vi "总磷总氮测量数据储存.vi"   [LabVIEW 2016, in "斯坦道总磷.lvlib"]
types:
  T1 = enum16{"水样测试", "标样核查", "跨度核查", "零点核查", "加标回收", "空白测试", "平行样"}
  T2 = cluster{"时间标识":timestamp, "测量模式":enum16{"维护数据", "水样测试", "标样核查", "零点核查", "跨度核查", "空白测试", "平行样测试", "加标回收", "空白校准", "标样校准", "初始化（清洗）", "快捷测试"}, "数据标记表":string, "监测值":sgl, "单位":u16, "数据标识":string, "因子编码":u32, "标样参考值":sgl, "F0":sgl, "F1":sgl, "F2":sgl, "F3":sgl, "F4":sgl, "F5":sgl, "F6":sgl, "F7":sgl, "X":sgl, "温度":sgl, "湿度":sgl, "量程标识":string, "SN":string, "跨度值":sgl, "X1":sgl}
  T3 = enum16{"维护数据", "水样测试", "标样核查", "零点核查", "跨度核查", "空白测试", "平行样测试", "加标回收", "空白校准", "标样校准", "初始化（清洗）", "快捷测试"}
  T4 = enum16{"维护数据", "水样测试", "标样核查", "零点核查", "跨度核查", "空白测试", "平行样测试", "加标回收", "空白校准", "标样校准", "初始化（清洗）"}
  T5 = cluster{"系统时间":timestamp, "工作状态":u16, "测量模式":enum16{"待机", "连续模式", "周期模式", "定点模式", "受控模式", "手动模式"}, "告警代码":u16, "故障代码":u16, "日志代码":u16, "软件版本":u16, "F0":sgl, "F1":sgl, "F2":sgl, "F3":sgl, "T":sgl, "H":sgl, "id":u16, "flowid":u16, "量程":u16, "总磷控温温度1":sgl, "营养盐控温温度2":sgl, "ADC":sgl}
  T6 = cluster{"运行模式":enum16{"维护模式", "常规模式", "应急模式", "质控模式"}, "质控频次":enum16{"关闭", "每天", "星期一", "星期二", "星期三", "星期四", "星期五", "星期六", "星期日"}, "空白核查时间":u16, "跨度核查时间":u16, "24H周期设置":bool[]}
  T7 = cluster{"因子编码":u32, "单位":u16, "标样参考值":sgl, "水样数据时间":timestamp, "水样实测值":sgl, "水样数据标识":string, "标样数据时间":timestamp, "标样实测值":sgl, "标样数据标识":string, "空白数据时间":timestamp, "空白实测值":sgl, "空白数据标识":string, "零点核查数据时间":timestamp, "零点核查实测值":sgl, "零点核查数据标识":string, "跨度核查数据时间":timestamp, "跨度核查实测值":sgl, "跨度核查数据标识":string, "加标回收数据时间":timestamp, "加标回收实测值":sgl, "加标回收数据标识":string, "平行样数据时间":timestamp, "平行样实测值":sgl, "平行样数据标识":string, "F0":sgl, "F1":sgl, "F2":sgl, "F3":sgl, "F4":sgl, "F5":sgl, "F6":sgl, "F7":sgl, "温度":sgl, "湿度":sgl, "X值":sgl, "fidrange":u16, "X1值":sgl}[]
  T8 = cluster{"因子编码":u32, "单位":u16, "标样参考值":sgl, "水样数据时间":timestamp, "水样实测值":sgl, "水样数据标识":string, "标样数据时间":timestamp, "标样实测值":sgl, "标样数据标识":string, "空白数据时间":timestamp, "空白实测值":sgl, "空白数据标识":string, "零点核查数据时间":timestamp, "零点核查实测值":sgl, "零点核查数据标识":string, "跨度核查数据时间":timestamp, "跨度核查实测值":sgl, "跨度核查数据标识":string, "加标回收数据时间":timestamp, "加标回收实测值":sgl, "加标回收数据标识":string, "平行样数据时间":timestamp, "平行样实测值":sgl, "平行样数据标识":string, "F0":sgl, "F1":sgl, "F2":sgl, "F3":sgl, "F4":sgl, "F5":sgl, "F6":sgl, "F7":sgl, "温度":sgl, "湿度":sgl, "X值":sgl, "fidrange":u16, "X1值":sgl}
  T9 = cluster{"总磷跨度值":dbl, "总磷零点标准液浓度":dbl, "总磷跨度标准液浓度":dbl, "总磷标准液标准浓度":dbl, "总氮跨度值":dbl, "总氮零点标准液浓度":dbl, "总氮跨度标准液浓度":dbl, "总氮标准液标准浓度":dbl, "COD跨度值":dbl, "COD零点标准液浓度":dbl, "COD跨度标准液浓度":dbl, "COD标准液标准浓度":dbl, "氨氮跨度值":dbl, "氨氮零点标准液浓度":dbl, "氨氮跨度标准液浓度":dbl, "氨氮标准液标准浓度":dbl, "磷酸盐跨度值":dbl, "磷酸盐零点标准液浓度":dbl, "磷酸盐跨度标准液浓度":dbl, "磷酸盐标准液标准浓度":dbl, "硝氮跨度值":dbl, "硝氮零点标准液浓度":dbl, "硝氮跨度标准液浓度":dbl, "硝氮标准液标准浓度":dbl, "亚硝氮跨度值":dbl, "亚硝氮零点标准液浓度":dbl, "亚硝氮跨度标准液浓度":dbl, "亚硝氮标准液标准浓度":dbl, "硫化物跨度值":dbl, "硫化物零点标准液浓度":dbl, "硫化物跨度标准液浓度":dbl, "硫化物标准液标准浓度":dbl, "硅酸盐跨度值":dbl, "硅酸盐零点标准液浓度":dbl, "硅酸盐跨度标准液浓度":dbl, "硅酸盐标准液标准浓度":dbl}
  T10 = typedef "斯坦道总磷.lvlib/关键参数.ctl" = cluster{"测量量程":sgl, "测量检出限":sgl, "测量精度":sgl, "测量间隔":sgl, "消解温度":sgl, "消解时长":sgl, "三项式系数":sgl, "二次多项式系数":sgl, "曲线斜率":sgl, "曲线截距":sgl, "线性相关系数":sgl, "空白校准时间":timestamp, "标样校准时间":timestamp, "测量信号值":sgl, "稀释倍数":sgl, "空白标定系数":sgl, "量程系数":sgl}
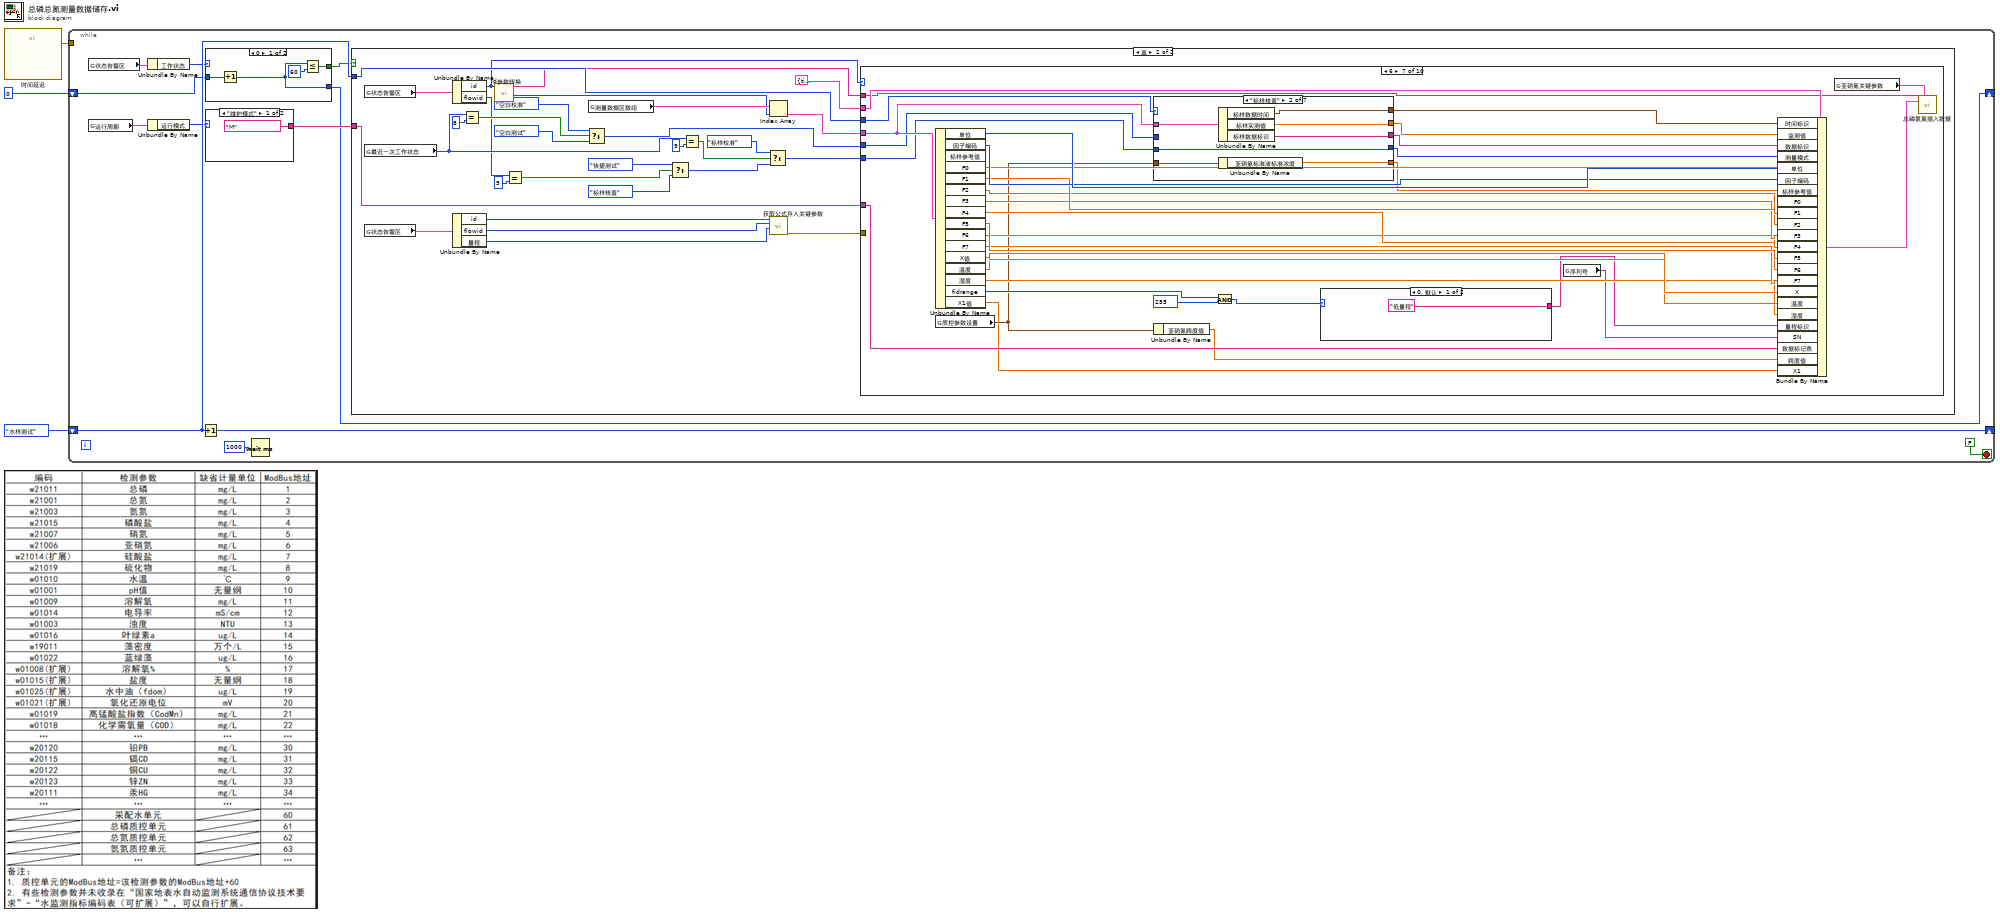
[diagram p0: block diagram]
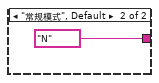
[diagram p3: hidden frame]
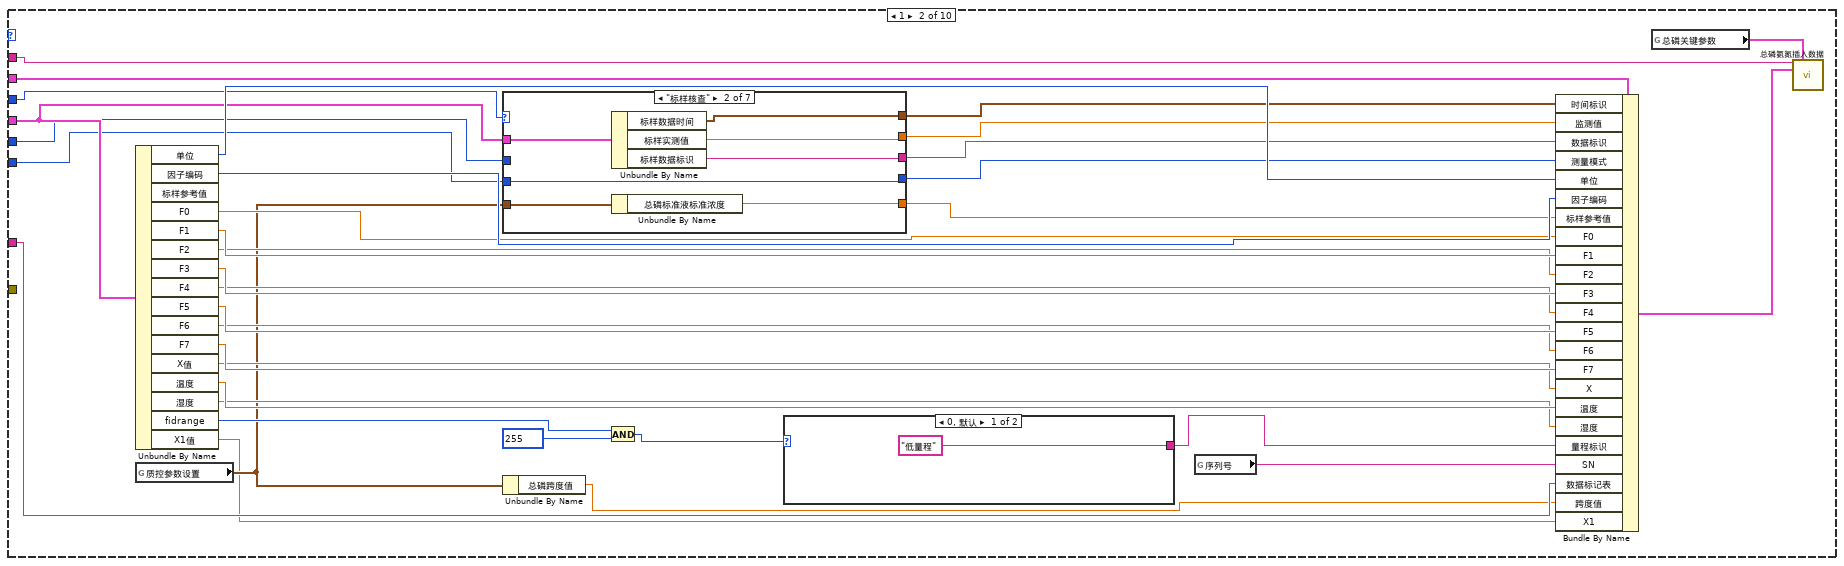
[diagram p6: hidden frame]
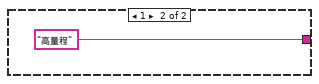
[diagram p7: hidden frame]
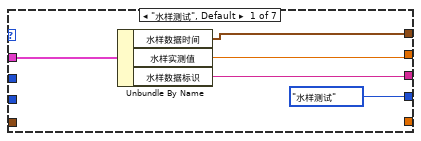
[diagram p8: hidden frame]
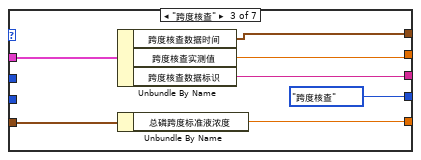
[diagram p9: hidden frame]
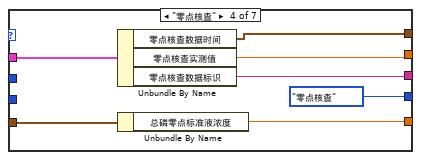
[diagram p10: hidden frame]
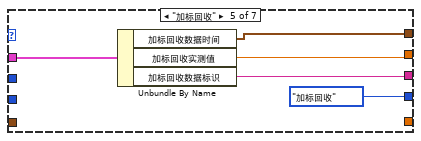
[diagram p11: hidden frame]
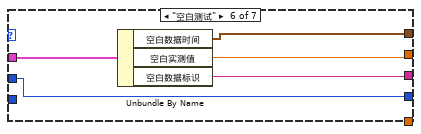
[diagram p12: hidden frame]
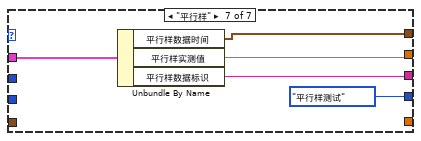
[diagram p13: hidden frame]
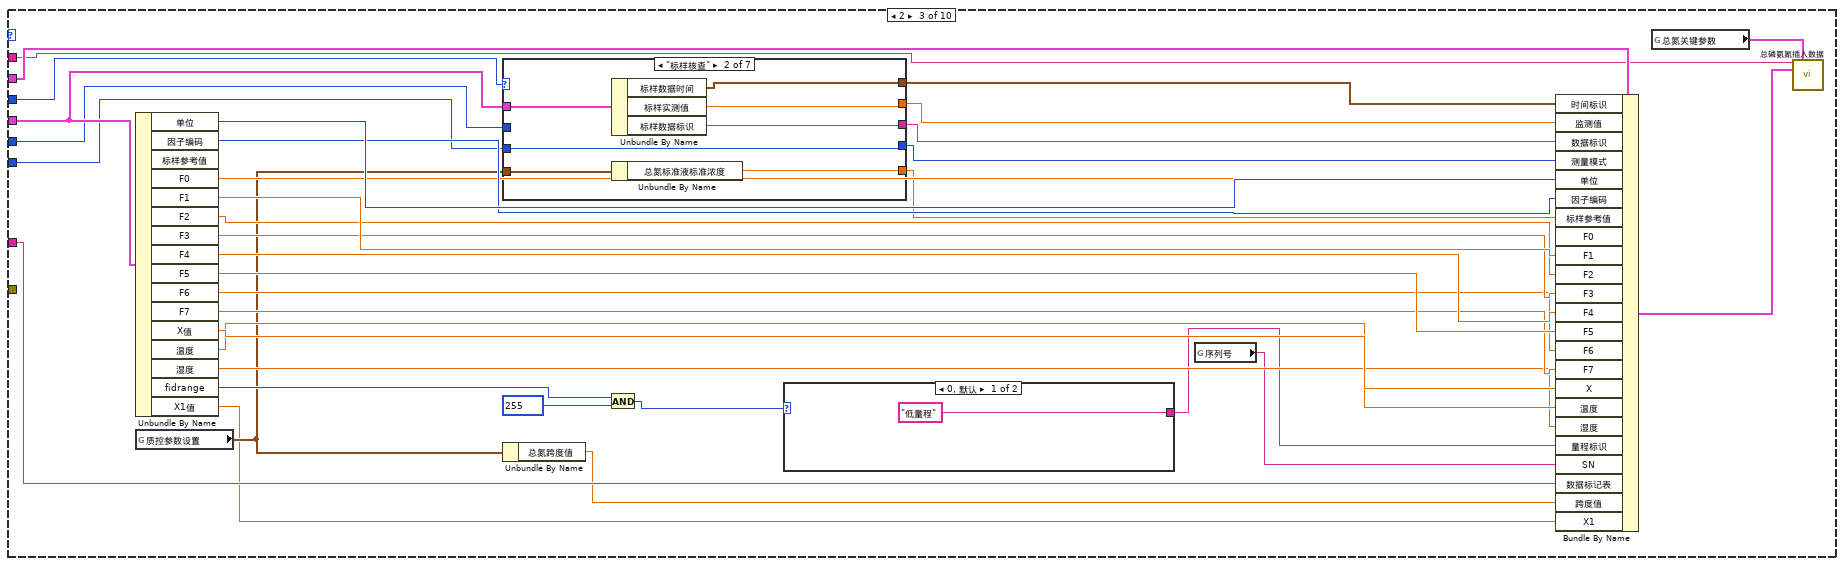
[diagram p14: hidden frame]
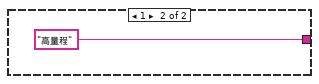
[diagram p15: hidden frame]
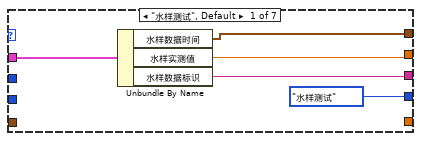
[diagram p16: hidden frame]
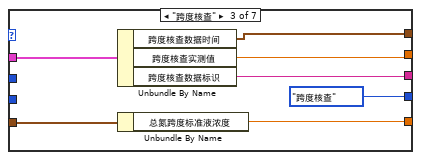
[diagram p17: hidden frame]
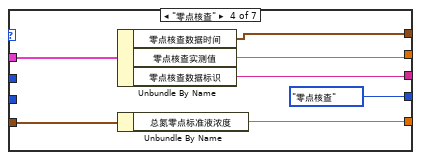
[diagram p18: hidden frame]
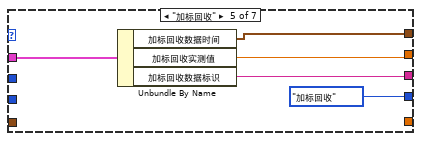
[diagram p19: hidden frame]
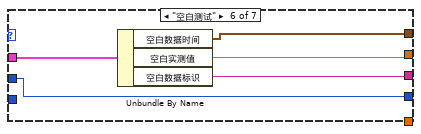
[diagram p20: hidden frame]
diagram:
  n1 = call "时间延迟"() -> ("error out"=w1:errorcluster)  [unwired: 11 in]
  n2 = while {
    shift-right: [w13] -> _
    shift-left: T1."水样测试" ("测量模式") -> [w12]
    shift-right: [w6] -> _
    shift-left: u32 0 ("等待时间（毫秒）") -> [w7]
    tunnel: w1 -> [_]
    stop <- FALSE stop-if-true
    n3 = global read "VAR总磷总氮全局变量.vi" "状态告警区"() -> (w9:T5)
    n4 = global read "总磷总氮断电保存全局变量.vi" "运行周期"() -> (w11:T6)
    n5 = Unbundle By Name(w9) -> ("工作状态"=w8:u16)
    n6 = Unbundle By Name(w11) -> ("运行模式"=w10:enum16{"维护模式", "常规模式", "应急模式", "质控模式"})
    n7 = Increment(x=w12) -> (x+1=w13:T1)
    n8 = case shown="0" w8 {
      tunnel: w7 -> [w19 _]
      tunnel: [w18 _] -> w6
      tunnel: [w16 _] -> w5
      frame 0 {
        n9 = Increment(x=w19) -> (x+1=w18:u32)
        n10 = Less Or Equal?(x=w18, y=u32 60) -> (x <= y?=w16:bool)
      }
      frame 1, Default {
      }
    }
    n11 = case shown="\"维护模式\"" w10 {
      tunnel: ["M" ("数据标记表") "N" ("数据标记表")] -> w14
      frame "维护模式" {
      }
      frame "常规模式", Default {
      }
    }
    n12 = Wait (ms)(milliseconds to wait=u32 1000 ("等待时间（毫秒）")) -> ()  [unwired: 1 out]
    n13 = case shown="真" w5 {
      tunnel: w14 -> [_ w51]
      tunnel: w12 -> [_ w50]
      frame False {
      }
      frame True {
        n14 = global read "VAR总磷总氮全局变量.vi" "状态告警区"() -> (w49:T5)
        n15 = global read "VAR总磷总氮全局变量.vi" "最近一次工作状态"() -> (w36:u16)
        n16 = global read "VAR总磷总氮全局变量.vi" "状态告警区"() -> (w26:T5)
        n17 = Unbundle By Name(w49) -> ("id"=w46:u16, "flowid"=w33:u16)
        n18 = Unbundle By Name(w26) -> ("id"=w22:u16, "flowid"=w25:u16, "量程"=w24:u16)
        n19 = Equal?(x=w36, y=u16 8) -> (x = y?=w42:bool)
        n20 = call "id参数转换.vi"("id"=w46) -> ("table输出"=w45:string, "数组资源索引"=w44:i32)  [unwired: 9 in]
        n21 = Equal?(x=w33, y=u16 5) -> (x = y?=w31:bool)
        n22 = Select(t=T3."空白校准" ("测量模式"), s=w42, f=T3."空白测试" ("测量模式")) -> (s? t:f=w35:T3)
        n23 = global read "VAR总磷总氮全局变量.vi" "测量数据区数组"() -> (w48:T7)
        n24 = Select(t=T3."快捷测试" ("测量模式"), s=w31, f=T3."标样核查" ("测量模式")) -> (s? t:f=w28:T3)
        n25 = Equal?(x=w36, y=u16 9) -> (x = y?=w38:bool)
        n26 = Select(t=T3."标样校准" ("测量模式"), s=w38, f=w28) -> (s? t:f=w34:T3)
        n27 = Index Array(array=w48, index=w44) -> (element=w47:T8)
        n28 = call "获取公式存入关键参数.vi"("量程"=w24, "flowid"=w25, "id"=w22) -> ("error out"=w23:errorcluster)  [unwired: 8 in]
        n29 = case shown="6" w46 {
          tunnel: w51 -> [_ w62 w140 w219 w297 w375 w453 w531 w609 w687]
          tunnel: w50 -> [_ w70 w151 w229 w307 w385 w463 w541 w619 w697]
          tunnel: T2 {"时间标识"=timestamp(0 s since 1904-01-01), "测量模式"=enum."水样测试", "数据标记表"="N", "监测值"=0.0, "单位"=0, "数据标识"="", "因子编码"=0, "标样参考值"=0.0, "F0"=0.0, "F1"=0.0, "F2"=0.0, "F3"=0.0, "F4"=0.0, "F5"=0.0, "F6"=0.0, "F7"=0.0, "X"=0.0, "温度"=0.0, "湿度"=0.0, "量程标识"="", "SN"="", "跨度值"=0.0, "X1"=0.0} ("data") -> [_ w60 w138 w217 w295 w373 w451 w529 w607 w685]
          tunnel: w47 -> [_ w57 w135 w214 w292 w370 w448 w526 w604 w681]
          tunnel: w45 -> [_ w56 w134 w212 w290 w368 w446 w524 w602 w680]
          tunnel: w35 -> [_ w55 w133 w210 w289 w367 w445 w522 w601 w679]
          tunnel: w34 -> [_ w54 w132 w211 w288 w366 w444 w523 w600 w678]
          tunnel: w23 -> [_ _ _ _ _ _ _ _ _ _]
          frame Default {
          }
          frame 1 {
            n30 = Unbundle By Name(w57) -> ("单位"=w86:u16, "因子编码"=w85:u32, "F0"=w84:sgl, "F1"=w83:sgl, "F2"=w82:sgl, "F3"=w81:sgl, "F4"=w80:sgl, "F5"=w79:sgl, "F6"=w78:sgl, "F7"=w77:sgl, "X值"=w76:sgl, "温度"=w75:sgl, "湿度"=w74:sgl, "fidrange"=w68:u16, "X1值"=w52:sgl)  [unwired: 1 out]
            n31 = global read "总磷总氮断电保存全局变量.vi" "质控参数设置"() -> (w59:T9)
            n32 = case shown="\"标样核查\"" w70 {
              tunnel: w57 -> [w93 w100 w107 w114 w119 w124 w129]
              tunnel: [w92 w99 w106 w113 w118 w123 w128] -> w71
              tunnel: [w91 w98 w105 w112 w117 w122 w127] -> w72
              tunnel: [w90 w97 w104 w111 w116 w121 w126] -> w73
              tunnel: [T4."水样测试" ("测量模式") w94 T4."跨度核查" ("测量模式") T4."零点核查" ("测量模式") T4."加标回收" ("测量模式") w120 T4."平行样测试" ("测量模式")] -> w61
              tunnel: w59 -> [_ w96 w102 w109 _ _ _]
              tunnel: [_ w95 w101 w108 _ _ _] -> w69
              tunnel: w55 -> [_ _ _ _ _ w120 _]
              tunnel: w54 -> [_ w94 _ _ _ _ _]
              frame "水样测试", Default {
                n33 = Unbundle By Name(w93) -> ("水样数据时间"=w92:timestamp, "水样实测值"=w91:sgl, "水样数据标识"=w90:string)
              }
              frame "标样核查" {
                n34 = Unbundle By Name(w100) -> ("标样数据时间"=w99:timestamp, "标样实测值"=w98:sgl, "标样数据标识"=w97:string)
                n35 = Unbundle By Name(w96) -> ("总磷标准液标准浓度"=w95:dbl)
              }
              frame "跨度核查" {
                n36 = Unbundle By Name(w107) -> ("跨度核查数据时间"=w106:timestamp, "跨度核查实测值"=w105:sgl, "跨度核查数据标识"=w104:string)
                n37 = Unbundle By Name(w102) -> ("总磷跨度标准液浓度"=w101:dbl)
              }
              frame "零点核查" {
                n38 = Unbundle By Name(w114) -> ("零点核查数据时间"=w113:timestamp, "零点核查实测值"=w112:sgl, "零点核查数据标识"=w111:string)
                n39 = Unbundle By Name(w109) -> ("总磷零点标准液浓度"=w108:dbl)
              }
              frame "加标回收" {
                n40 = Unbundle By Name(w119) -> ("加标回收数据时间"=w118:timestamp, "加标回收实测值"=w117:sgl, "加标回收数据标识"=w116:string)
              }
              frame "空白测试" {
                n41 = Unbundle By Name(w124) -> ("空白数据时间"=w123:timestamp, "空白实测值"=w122:sgl, "空白数据标识"=w121:string)
              }
              frame "平行样" {
                n42 = Unbundle By Name(w129) -> ("平行样数据时间"=w128:timestamp, "平行样实测值"=w127:sgl, "平行样数据标识"=w126:string)
              }
            }
            n43 = Unbundle By Name(w59) -> ("总磷跨度值"=w58:dbl)
            n44 = And(x=w68, y=u16 255) -> (x .and. y?=w66:u16)
            n45 = case shown="0, 默认" w66 {
              tunnel: ["低量程" ("格式字符串") "高量程" ("格式字符串")] -> w65
              frame 0, Default {
              }
              frame 1 {
              }
            }
            n46 = global read "VAR总磷总氮全局变量.vi" "序列号"() -> (w63:string)
            n47 = Bundle By Name(cluster=w60, "时间标识"=w71, "监测值"=w72, "数据标识"=w73, "测量模式"=w61, "单位"=w86, "因子编码"=w85, "标样参考值"=w69, "F0"=w84, "F1"=w83, "F2"=w82, "F3"=w81, "F4"=w80, "F5"=w79, "F6"=w78, "F7"=w77, "X"=w76, "温度"=w75, "湿度"=w74, "量程标识"=w65, "SN"=w63, "数据标记表"=w62, "跨度值"=w58, "X1"=w52) -> (w64:T2)
            n48 = global read "VAR总磷总氮全局变量.vi" "总磷关键参数"() -> (w53:T10)
            n49 = call "总磷氨氮插入数据.vi"("table"=w56, "关键参数"=w53, "data"=w64) -> ()  [unwired: 12 in, 1 out]
          }
          frame 2 {
            n50 = Unbundle By Name(w135) -> ("单位"=w164:u16, "因子编码"=w163:u32, "F0"=w162:sgl, "F1"=w161:sgl, "F2"=w160:sgl, "F3"=w159:sgl, "F4"=w158:sgl, "F5"=w157:sgl, "F6"=w156:sgl, "F7"=w155:sgl, "X值"=w154:sgl, "温度"=w153:sgl, "湿度"=w152:sgl, "fidrange"=w144:u16, "X1值"=w130:sgl)  [unwired: 1 out]
            n51 = global read "总磷总氮断电保存全局变量.vi" "质控参数设置"() -> (w137:T9)
            n52 = case shown="\"标样核查\"" w151 {
              tunnel: w135 -> [w171 w178 w185 w192 w197 w202 w207]
              tunnel: [w170 w177 w184 w191 w196 w201 w206] -> w150
              tunnel: [w169 w176 w183 w190 w195 w200 w205] -> w149
              tunnel: [w168 w175 w182 w189 w194 w199 w204] -> w148
              tunnel: [T4."水样测试" ("测量模式") w172 T4."跨度核查" ("测量模式") T4."零点核查" ("测量模式") T4."加标回收" ("测量模式") w198 T4."平行样测试" ("测量模式")] -> w139
              tunnel: w137 -> [_ w174 w180 w187 _ _ _]
              tunnel: [_ w173 w179 w186 _ _ _] -> w147
              tunnel: w133 -> [_ _ _ _ _ w198 _]
              tunnel: w132 -> [_ w172 _ _ _ _ _]
              frame "水样测试", Default {
                n53 = Unbundle By Name(w171) -> ("水样数据时间"=w170:timestamp, "水样实测值"=w169:sgl, "水样数据标识"=w168:string)
              }
              frame "标样核查" {
                n54 = Unbundle By Name(w178) -> ("标样数据时间"=w177:timestamp, "标样实测值"=w176:sgl, "标样数据标识"=w175:string)
                n55 = Unbundle By Name(w174) -> ("总氮标准液标准浓度"=w173:dbl)
              }
              frame "跨度核查" {
                n56 = Unbundle By Name(w185) -> ("跨度核查数据时间"=w184:timestamp, "跨度核查实测值"=w183:sgl, "跨度核查数据标识"=w182:string)
                n57 = Unbundle By Name(w180) -> ("总氮跨度标准液浓度"=w179:dbl)
              }
              frame "零点核查" {
                n58 = Unbundle By Name(w192) -> ("零点核查数据时间"=w191:timestamp, "零点核查实测值"=w190:sgl, "零点核查数据标识"=w189:string)
                n59 = Unbundle By Name(w187) -> ("总氮零点标准液浓度"=w186:dbl)
              }
              frame "加标回收" {
                n60 = Unbundle By Name(w197) -> ("加标回收数据时间"=w196:timestamp, "加标回收实测值"=w195:sgl, "加标回收数据标识"=w194:string)
              }
              frame "空白测试" {
                n61 = Unbundle By Name(w202) -> ("空白数据时间"=w201:timestamp, "空白实测值"=w200:sgl, "空白数据标识"=w199:string)
              }
              frame "平行样" {
                n62 = Unbundle By Name(w207) -> ("平行样数据时间"=w206:timestamp, "平行样实测值"=w205:sgl, "平行样数据标识"=w204:string)
              }
            }
            n63 = Unbundle By Name(w137) -> ("总氮跨度值"=w136:dbl)
            n64 = And(x=w144, y=u16 255) -> (x .and. y?=w145:u16)
            n65 = case shown="0, 默认" w145 {
              tunnel: ["低量程" ("格式字符串") "高量程" ("格式字符串")] -> w143
              frame 0, Default {
              }
              frame 1 {
              }
            }
            n66 = global read "VAR总磷总氮全局变量.vi" "序列号"() -> (w141:string)
            n67 = Bundle By Name(cluster=w138, "时间标识"=w150, "监测值"=w149, "数据标识"=w148, "测量模式"=w139, "单位"=w164, "因子编码"=w163, "标样参考值"=w147, "F0"=w162, "F1"=w161, "F2"=w160, "F3"=w159, "F4"=w158, "F5"=w157, "F6"=w156, "F7"=w155, "X"=w154, "温度"=w153, "湿度"=w152, "量程标识"=w143, "SN"=w141, "数据标记表"=w140, "跨度值"=w136, "X1"=w130) -> (w142:T2)
            n68 = global read "VAR总磷总氮全局变量.vi" "总氮关键参数"() -> (w131:T10)
            n69 = call "总磷氨氮插入数据.vi"("table"=w134, "关键参数"=w131, "data"=w142) -> ()  [unwired: 12 in, 1 out]
          }
          frame 3 {
            n70 = Unbundle By Name(w214) -> ("单位"=w242:u16, "因子编码"=w241:u32, "F0"=w240:sgl, "F1"=w239:sgl, "F2"=w238:sgl, "F3"=w237:sgl, "F4"=w236:sgl, "F5"=w235:sgl, "F6"=w234:sgl, "F7"=w233:sgl, "X值"=w232:sgl, "温度"=w231:sgl, "湿度"=w230:sgl, "fidrange"=w222:u16, "X1值"=w208:sgl)  [unwired: 1 out]
            n71 = global read "总磷总氮断电保存全局变量.vi" "质控参数设置"() -> (w216:T9)
            n72 = case shown="\"空白测试\"" w229 {
              tunnel: w214 -> [w249 w256 w263 w270 w275 w280 w285]
              tunnel: [w248 w255 w262 w269 w274 w279 w284] -> w228
              tunnel: [w247 w254 w261 w268 w273 w278 w283] -> w227
              tunnel: [w246 w253 w260 w267 w272 w277 w282] -> w226
              tunnel: [T4."水样测试" ("测量模式") w250 T4."跨度核查" ("测量模式") T4."零点核查" ("测量模式") T4."加标回收" ("测量模式") w276 T4."平行样测试" ("测量模式")] -> w218
              tunnel: w216 -> [_ w252 w258 w265 _ _ _]
              tunnel: [_ w251 w257 w264 _ _ _] -> w225
              tunnel: w211 -> [_ w250 _ _ _ _ _]
              tunnel: w210 -> [_ _ _ _ _ w276 _]
              frame "水样测试", Default {
                n73 = Unbundle By Name(w249) -> ("水样数据时间"=w248:timestamp, "水样实测值"=w247:sgl, "水样数据标识"=w246:string)
              }
              frame "标样核查" {
                n74 = Unbundle By Name(w256) -> ("标样数据时间"=w255:timestamp, "标样实测值"=w254:sgl, "标样数据标识"=w253:string)
                n75 = Unbundle By Name(w252) -> ("氨氮标准液标准浓度"=w251:dbl)
              }
              frame "跨度核查" {
                n76 = Unbundle By Name(w263) -> ("跨度核查数据时间"=w262:timestamp, "跨度核查实测值"=w261:sgl, "跨度核查数据标识"=w260:string)
                n77 = Unbundle By Name(w258) -> ("氨氮跨度标准液浓度"=w257:dbl)
              }
              frame "零点核查" {
                n78 = Unbundle By Name(w270) -> ("零点核查数据时间"=w269:timestamp, "零点核查实测值"=w268:sgl, "零点核查数据标识"=w267:string)
                n79 = Unbundle By Name(w265) -> ("氨氮零点标准液浓度"=w264:dbl)
              }
              frame "加标回收" {
                n80 = Unbundle By Name(w275) -> ("加标回收数据时间"=w274:timestamp, "加标回收实测值"=w273:sgl, "加标回收数据标识"=w272:string)
              }
              frame "空白测试" {
                n81 = Unbundle By Name(w280) -> ("空白数据时间"=w279:timestamp, "空白实测值"=w278:sgl, "空白数据标识"=w277:string)
              }
              frame "平行样" {
                n82 = Unbundle By Name(w285) -> ("平行样数据时间"=w284:timestamp, "平行样实测值"=w283:sgl, "平行样数据标识"=w282:string)
              }
            }
            n83 = Unbundle By Name(w216) -> ("氨氮跨度值"=w215:dbl)
            n84 = And(x=w222, y=u16 255) -> (x .and. y?=w223:u16)
            n85 = case shown="0, 默认" w223 {
              tunnel: ["低量程" ("格式字符串") "高量程" ("格式字符串")] -> w221
              frame 0, Default {
              }
              frame 1 {
              }
            }
            n86 = global read "VAR总磷总氮全局变量.vi" "序列号"() -> (w220:string)
            n87 = Bundle By Name(cluster=w217, "时间标识"=w228, "监测值"=w227, "数据标识"=w226, "测量模式"=w218, "单位"=w242, "因子编码"=w241, "标样参考值"=w225, "F0"=w240, "F1"=w239, "F2"=w238, "F3"=w237, "F4"=w236, "F5"=w235, "F6"=w234, "F7"=w233, "X"=w232, "温度"=w231, "湿度"=w230, "量程标识"=w221, "SN"=w220, "数据标记表"=w219, "跨度值"=w215, "X1"=w208) -> (w213:T2)
            n88 = global read "VAR总磷总氮全局变量.vi" "氨氮关键参数"() -> (w209:T10)
            n89 = call "总磷氨氮插入数据.vi"("table"=w212, "关键参数"=w209, "data"=w213) -> ()  [unwired: 12 in, 1 out]
          }
          frame 4 {
            n90 = Unbundle By Name(w292) -> ("单位"=w320:u16, "因子编码"=w319:u32, "F0"=w318:sgl, "F1"=w317:sgl, "F2"=w316:sgl, "F3"=w315:sgl, "F4"=w314:sgl, "F5"=w313:sgl, "F6"=w312:sgl, "F7"=w311:sgl, "X值"=w310:sgl, "温度"=w309:sgl, "湿度"=w308:sgl, "fidrange"=w300:u16, "X1值"=w286:sgl)  [unwired: 1 out]
            n91 = global read "总磷总氮断电保存全局变量.vi" "质控参数设置"() -> (w294:T9)
            n92 = case shown="\"标样核查\"" w307 {
              tunnel: w292 -> [w327 w334 w341 w348 w353 w358 w363]
              tunnel: [w326 w333 w340 w347 w352 w357 w362] -> w306
              tunnel: [w325 w332 w339 w346 w351 w356 w361] -> w305
              tunnel: [w324 w331 w338 w345 w350 w355 w360] -> w304
              tunnel: [T4."水样测试" ("测量模式") w328 T4."跨度核查" ("测量模式") T4."零点核查" ("测量模式") T4."加标回收" ("测量模式") w354 T4."平行样测试" ("测量模式")] -> w296
              tunnel: w294 -> [_ w330 w336 w343 _ _ _]
              tunnel: [_ w329 w335 w342 _ _ _] -> w303
              tunnel: w289 -> [_ _ _ _ _ w354 _]
              tunnel: w288 -> [_ w328 _ _ _ _ _]
              frame "水样测试", Default {
                n93 = Unbundle By Name(w327) -> ("水样数据时间"=w326:timestamp, "水样实测值"=w325:sgl, "水样数据标识"=w324:string)
              }
              frame "标样核查" {
                n94 = Unbundle By Name(w334) -> ("标样数据时间"=w333:timestamp, "标样实测值"=w332:sgl, "标样数据标识"=w331:string)
                n95 = Unbundle By Name(w330) -> ("磷酸盐标准液标准浓度"=w329:dbl)
              }
              frame "跨度核查" {
                n96 = Unbundle By Name(w341) -> ("跨度核查数据时间"=w340:timestamp, "跨度核查实测值"=w339:sgl, "跨度核查数据标识"=w338:string)
                n97 = Unbundle By Name(w336) -> ("磷酸盐跨度标准液浓度"=w335:dbl)
              }
              frame "零点核查" {
                n98 = Unbundle By Name(w348) -> ("零点核查数据时间"=w347:timestamp, "零点核查实测值"=w346:sgl, "零点核查数据标识"=w345:string)
                n99 = Unbundle By Name(w343) -> ("磷酸盐零点标准液浓度"=w342:dbl)
              }
              frame "加标回收" {
                n100 = Unbundle By Name(w353) -> ("加标回收数据时间"=w352:timestamp, "加标回收实测值"=w351:sgl, "加标回收数据标识"=w350:string)
              }
              frame "空白测试" {
                n101 = Unbundle By Name(w358) -> ("空白数据时间"=w357:timestamp, "空白实测值"=w356:sgl, "空白数据标识"=w355:string)
              }
              frame "平行样" {
                n102 = Unbundle By Name(w363) -> ("平行样数据时间"=w362:timestamp, "平行样实测值"=w361:sgl, "平行样数据标识"=w360:string)
              }
            }
            n103 = Unbundle By Name(w294) -> ("磷酸盐跨度值"=w293:dbl)
            n104 = And(x=w300, y=u16 255) -> (x .and. y?=w301:u16)
            n105 = case shown="0, 默认" w301 {
              tunnel: ["低量程" ("格式字符串") "高量程" ("格式字符串")] -> w299
              frame 0, Default {
              }
              frame 1 {
              }
            }
            n106 = global read "VAR总磷总氮全局变量.vi" "序列号"() -> (w298:string)
            n107 = Bundle By Name(cluster=w295, "时间标识"=w306, "监测值"=w305, "数据标识"=w304, "测量模式"=w296, "单位"=w320, "因子编码"=w319, "标样参考值"=w303, "F0"=w318, "F1"=w317, "F2"=w316, "F3"=w315, "F4"=w314, "F5"=w313, "F6"=w312, "F7"=w311, "X"=w310, "温度"=w309, "湿度"=w308, "量程标识"=w299, "SN"=w298, "数据标记表"=w297, "跨度值"=w293, "X1"=w286) -> (w291:T2)
            n108 = global read "VAR总磷总氮全局变量.vi" "磷酸盐关键参数"() -> (w287:T10)
            n109 = call "总磷氨氮插入数据.vi"("table"=w290, "关键参数"=w287, "data"=w291) -> ()  [unwired: 12 in, 1 out]
          }
          frame 5 {
            n110 = Unbundle By Name(w370) -> ("单位"=w398:u16, "因子编码"=w397:u32, "F0"=w396:sgl, "F1"=w395:sgl, "F2"=w394:sgl, "F3"=w393:sgl, "F4"=w392:sgl, "F5"=w391:sgl, "F6"=w390:sgl, "F7"=w389:sgl, "X值"=w388:sgl, "温度"=w387:sgl, "湿度"=w386:sgl, "fidrange"=w378:u16, "X1值"=w364:sgl)  [unwired: 1 out]
            n111 = global read "总磷总氮断电保存全局变量.vi" "质控参数设置"() -> (w372:T9)
            n112 = case shown="\"标样核查\"" w385 {
              tunnel: w370 -> [w405 w412 w419 w426 w431 w436 w441]
              tunnel: [w404 w411 w418 w425 w430 w435 w440] -> w384
              tunnel: [w403 w410 w417 w424 w429 w434 w439] -> w383
              tunnel: [w402 w409 w416 w423 w428 w433 w438] -> w382
              tunnel: [T4."水样测试" ("测量模式") w406 T4."跨度核查" ("测量模式") T4."零点核查" ("测量模式") T4."加标回收" ("测量模式") w432 T4."平行样测试" ("测量模式")] -> w374
              tunnel: w372 -> [_ w408 w414 w421 _ _ _]
              tunnel: [_ w407 w413 w420 _ _ _] -> w381
              tunnel: w367 -> [_ _ _ _ _ w432 _]
              tunnel: w366 -> [_ w406 _ _ _ _ _]
              frame "水样测试", Default {
                n113 = Unbundle By Name(w405) -> ("水样数据时间"=w404:timestamp, "水样实测值"=w403:sgl, "水样数据标识"=w402:string)
              }
              frame "标样核查" {
                n114 = Unbundle By Name(w412) -> ("标样数据时间"=w411:timestamp, "标样实测值"=w410:sgl, "标样数据标识"=w409:string)
                n115 = Unbundle By Name(w408) -> ("硝氮标准液标准浓度"=w407:dbl)
              }
              frame "跨度核查" {
                n116 = Unbundle By Name(w419) -> ("跨度核查数据时间"=w418:timestamp, "跨度核查实测值"=w417:sgl, "跨度核查数据标识"=w416:string)
                n117 = Unbundle By Name(w414) -> ("硝氮跨度标准液浓度"=w413:dbl)
              }
              frame "零点核查" {
                n118 = Unbundle By Name(w426) -> ("零点核查数据时间"=w425:timestamp, "零点核查实测值"=w424:sgl, "零点核查数据标识"=w423:string)
                n119 = Unbundle By Name(w421) -> ("硝氮零点标准液浓度"=w420:dbl)
              }
              frame "加标回收" {
                n120 = Unbundle By Name(w431) -> ("加标回收数据时间"=w430:timestamp, "加标回收实测值"=w429:sgl, "加标回收数据标识"=w428:string)
              }
              frame "空白测试" {
                n121 = Unbundle By Name(w436) -> ("空白数据时间"=w435:timestamp, "空白实测值"=w434:sgl, "空白数据标识"=w433:string)
              }
              frame "平行样" {
                n122 = Unbundle By Name(w441) -> ("平行样数据时间"=w440:timestamp, "平行样实测值"=w439:sgl, "平行样数据标识"=w438:string)
              }
            }
            n123 = Unbundle By Name(w372) -> ("硝氮跨度值"=w371:dbl)
            n124 = And(x=w378, y=u16 255) -> (x .and. y?=w379:u16)
            n125 = case shown="0, 默认" w379 {
              tunnel: ["低量程" ("格式字符串") "高量程" ("格式字符串")] -> w377
              frame 0, Default {
              }
              frame 1 {
              }
            }
            n126 = global read "VAR总磷总氮全局变量.vi" "序列号"() -> (w376:string)
            n127 = Bundle By Name(cluster=w373, "时间标识"=w384, "监测值"=w383, "数据标识"=w382, "测量模式"=w374, "单位"=w398, "因子编码"=w397, "标样参考值"=w381, "F0"=w396, "F1"=w395, "F2"=w394, "F3"=w393, "F4"=w392, "F5"=w391, "F6"=w390, "F7"=w389, "X"=w388, "温度"=w387, "湿度"=w386, "量程标识"=w377, "SN"=w376, "数据标记表"=w375, "跨度值"=w371, "X1"=w364) -> (w369:T2)
            n128 = global read "VAR总磷总氮全局变量.vi" "硝氮关键参数"() -> (w365:T10)
            n129 = call "总磷氨氮插入数据.vi"("table"=w368, "关键参数"=w365, "data"=w369) -> ()  [unwired: 12 in, 1 out]
          }
          frame 6 {
            n130 = Unbundle By Name(w448) -> ("单位"=w476:u16, "因子编码"=w475:u32, "F0"=w474:sgl, "F1"=w473:sgl, "F2"=w472:sgl, "F3"=w471:sgl, "F4"=w470:sgl, "F5"=w469:sgl, "F6"=w468:sgl, "F7"=w467:sgl, "X值"=w466:sgl, "温度"=w465:sgl, "湿度"=w464:sgl, "fidrange"=w456:u16, "X1值"=w442:sgl)  [unwired: 1 out]
            n131 = global read "总磷总氮断电保存全局变量.vi" "质控参数设置"() -> (w450:T9)
            n132 = case shown="\"标样核查\"" w463 {
              tunnel: w448 -> [w483 w490 w497 w504 w509 w514 w519]
              tunnel: [w482 w489 w496 w503 w508 w513 w518] -> w462
              tunnel: [w481 w488 w495 w502 w507 w512 w517] -> w461
              tunnel: [w480 w487 w494 w501 w506 w511 w516] -> w460
              tunnel: [T4."水样测试" ("测量模式") w484 T4."跨度核查" ("测量模式") T4."零点核查" ("测量模式") T4."加标回收" ("测量模式") w510 T4."平行样测试" ("测量模式")] -> w452
              tunnel: w450 -> [_ w486 w492 w499 _ _ _]
              tunnel: [_ w485 w491 w498 _ _ _] -> w459
              tunnel: w445 -> [_ _ _ _ _ w510 _]
              tunnel: w444 -> [_ w484 _ _ _ _ _]
              frame "水样测试", Default {
                n133 = Unbundle By Name(w483) -> ("水样数据时间"=w482:timestamp, "水样实测值"=w481:sgl, "水样数据标识"=w480:string)
              }
              frame "标样核查" {
                n134 = Unbundle By Name(w490) -> ("标样数据时间"=w489:timestamp, "标样实测值"=w488:sgl, "标样数据标识"=w487:string)
                n135 = Unbundle By Name(w486) -> ("亚硝氮标准液标准浓度"=w485:dbl)
              }
              frame "跨度核查" {
                n136 = Unbundle By Name(w497) -> ("跨度核查数据时间"=w496:timestamp, "跨度核查实测值"=w495:sgl, "跨度核查数据标识"=w494:string)
                n137 = Unbundle By Name(w492) -> ("亚硝氮跨度标准液浓度"=w491:dbl)
              }
              frame "零点核查" {
                n138 = Unbundle By Name(w504) -> ("零点核查数据时间"=w503:timestamp, "零点核查实测值"=w502:sgl, "零点核查数据标识"=w501:string)
                n139 = Unbundle By Name(w499) -> ("亚硝氮零点标准液浓度"=w498:dbl)
              }
              frame "加标回收" {
                n140 = Unbundle By Name(w509) -> ("加标回收数据时间"=w508:timestamp, "加标回收实测值"=w507:sgl, "加标回收数据标识"=w506:string)
              }
              frame "空白测试" {
                n141 = Unbundle By Name(w514) -> ("空白数据时间"=w513:timestamp, "空白实测值"=w512:sgl, "空白数据标识"=w511:string)
              }
              frame "平行样" {
                n142 = Unbundle By Name(w519) -> ("平行样数据时间"=w518:timestamp, "平行样实测值"=w517:sgl, "平行样数据标识"=w516:string)
              }
            }
            n143 = Unbundle By Name(w450) -> ("亚硝氮跨度值"=w449:dbl)
            n144 = And(x=w456, y=u16 255) -> (x .and. y?=w457:u16)
            n145 = case shown="0, 默认" w457 {
              tunnel: ["低量程" ("格式字符串") "高量程" ("格式字符串")] -> w455
              frame 0, Default {
              }
              frame 1 {
              }
            }
            n146 = global read "VAR总磷总氮全局变量.vi" "序列号"() -> (w454:string)
            n147 = Bundle By Name(cluster=w451, "时间标识"=w462, "监测值"=w461, "数据标识"=w460, "测量模式"=w452, "单位"=w476, "因子编码"=w475, "标样参考值"=w459, "F0"=w474, "F1"=w473, "F2"=w472, "F3"=w471, "F4"=w470, "F5"=w469, "F6"=w468, "F7"=w467, "X"=w466, "温度"=w465, "湿度"=w464, "量程标识"=w455, "SN"=w454, "数据标记表"=w453, "跨度值"=w449, "X1"=w442) -> (w447:T2)
            n148 = global read "VAR总磷总氮全局变量.vi" "亚硝氮关键参数"() -> (w443:T10)
            n149 = call "总磷氨氮插入数据.vi"("table"=w446, "关键参数"=w443, "data"=w447) -> ()  [unwired: 12 in, 1 out]
          }
          frame 7 {
            n150 = Unbundle By Name(w526) -> ("单位"=w554:u16, "因子编码"=w553:u32, "F0"=w552:sgl, "F1"=w551:sgl, "F2"=w550:sgl, "F3"=w549:sgl, "F4"=w548:sgl, "F5"=w547:sgl, "F6"=w546:sgl, "F7"=w545:sgl, "X值"=w544:sgl, "温度"=w543:sgl, "湿度"=w542:sgl, "fidrange"=w534:u16, "X1值"=w520:sgl)  [unwired: 1 out]
            n151 = global read "总磷总氮断电保存全局变量.vi" "质控参数设置"() -> (w528:T9)
            n152 = case shown="\"空白测试\"" w541 {
              tunnel: w526 -> [w561 w568 w575 w582 w587 w592 w597]
              tunnel: [w560 w567 w574 w581 w586 w591 w596] -> w540
              tunnel: [w559 w566 w573 w580 w585 w590 w595] -> w539
              tunnel: [w558 w565 w572 w579 w584 w589 w594] -> w538
              tunnel: [T4."水样测试" ("测量模式") w562 T4."跨度核查" ("测量模式") T4."零点核查" ("测量模式") T4."加标回收" ("测量模式") w588 T4."平行样测试" ("测量模式")] -> w530
              tunnel: w528 -> [_ w564 w570 w577 _ _ _]
              tunnel: [_ w563 w569 w576 _ _ _] -> w537
              tunnel: w523 -> [_ w562 _ _ _ _ _]
              tunnel: w522 -> [_ _ _ _ _ w588 _]
              frame "水样测试", Default {
                n153 = Unbundle By Name(w561) -> ("水样数据时间"=w560:timestamp, "水样实测值"=w559:sgl, "水样数据标识"=w558:string)
              }
              frame "标样核查" {
                n154 = Unbundle By Name(w568) -> ("标样数据时间"=w567:timestamp, "标样实测值"=w566:sgl, "标样数据标识"=w565:string)
                n155 = Unbundle By Name(w564) -> ("硅酸盐标准液标准浓度"=w563:dbl)
              }
              frame "跨度核查" {
                n156 = Unbundle By Name(w575) -> ("跨度核查数据时间"=w574:timestamp, "跨度核查实测值"=w573:sgl, "跨度核查数据标识"=w572:string)
                n157 = Unbundle By Name(w570) -> ("硅酸盐跨度标准液浓度"=w569:dbl)
              }
              frame "零点核查" {
                n158 = Unbundle By Name(w582) -> ("零点核查数据时间"=w581:timestamp, "零点核查实测值"=w580:sgl, "零点核查数据标识"=w579:string)
                n159 = Unbundle By Name(w577) -> ("硅酸盐零点标准液浓度"=w576:dbl)
              }
              frame "加标回收" {
                n160 = Unbundle By Name(w587) -> ("加标回收数据时间"=w586:timestamp, "加标回收实测值"=w585:sgl, "加标回收数据标识"=w584:string)
              }
              frame "空白测试" {
                n161 = Unbundle By Name(w592) -> ("空白数据时间"=w591:timestamp, "空白实测值"=w590:sgl, "空白数据标识"=w589:string)
              }
              frame "平行样" {
                n162 = Unbundle By Name(w597) -> ("平行样数据时间"=w596:timestamp, "平行样实测值"=w595:sgl, "平行样数据标识"=w594:string)
              }
            }
            n163 = Unbundle By Name(w528) -> ("硅酸盐跨度值"=w527:dbl)
            n164 = And(x=w534, y=u16 255) -> (x .and. y?=w535:u16)
            n165 = case shown="0, 默认" w535 {
              tunnel: ["低量程" ("格式字符串") "高量程" ("格式字符串")] -> w533
              frame 0, Default {
              }
              frame 1 {
              }
            }
            n166 = global read "VAR总磷总氮全局变量.vi" "序列号"() -> (w532:string)
            n167 = Bundle By Name(cluster=w529, "时间标识"=w540, "监测值"=w539, "数据标识"=w538, "测量模式"=w530, "单位"=w554, "因子编码"=w553, "标样参考值"=w537, "F0"=w552, "F1"=w551, "F2"=w550, "F3"=w549, "F4"=w548, "F5"=w547, "F6"=w546, "F7"=w545, "X"=w544, "温度"=w543, "湿度"=w542, "量程标识"=w533, "SN"=w532, "数据标记表"=w531, "跨度值"=w527, "X1"=w520) -> (w525:T2)
            n168 = global read "VAR总磷总氮全局变量.vi" "硅酸盐关键参数"() -> (w521:T10)
            n169 = call "总磷氨氮插入数据.vi"("table"=w524, "关键参数"=w521, "data"=w525) -> ()  [unwired: 12 in, 1 out]
          }
          frame 8 {
            n170 = Unbundle By Name(w604) -> ("单位"=w632:u16, "因子编码"=w631:u32, "F0"=w630:sgl, "F1"=w629:sgl, "F2"=w628:sgl, "F3"=w627:sgl, "F4"=w626:sgl, "F5"=w625:sgl, "F6"=w624:sgl, "F7"=w623:sgl, "X值"=w622:sgl, "温度"=w621:sgl, "湿度"=w620:sgl, "fidrange"=w612:u16, "X1值"=w598:sgl)  [unwired: 1 out]
            n171 = global read "总磷总氮断电保存全局变量.vi" "质控参数设置"() -> (w606:T9)
            n172 = case shown="\"标样核查\"" w619 {
              tunnel: w604 -> [w639 w646 w653 w660 w665 w670 w675]
              tunnel: [w638 w645 w652 w659 w664 w669 w674] -> w618
              tunnel: [w637 w644 w651 w658 w663 w668 w673] -> w617
              tunnel: [w636 w643 w650 w657 w662 w667 w672] -> w616
              tunnel: [T4."水样测试" ("测量模式") w640 T4."跨度核查" ("测量模式") T4."零点核查" ("测量模式") T4."加标回收" ("测量模式") w666 T4."平行样测试" ("测量模式")] -> w608
              tunnel: w606 -> [_ w642 w648 w655 _ _ _]
              tunnel: [_ w641 w647 w654 _ _ _] -> w615
              tunnel: w601 -> [_ _ _ _ _ w666 _]
              tunnel: w600 -> [_ w640 _ _ _ _ _]
              frame "水样测试", Default {
                n173 = Unbundle By Name(w639) -> ("水样数据时间"=w638:timestamp, "水样实测值"=w637:sgl, "水样数据标识"=w636:string)
              }
              frame "标样核查" {
                n174 = Unbundle By Name(w646) -> ("标样数据时间"=w645:timestamp, "标样实测值"=w644:sgl, "标样数据标识"=w643:string)
                n175 = Unbundle By Name(w642) -> ("硫化物标准液标准浓度"=w641:dbl)
              }
              frame "跨度核查" {
                n176 = Unbundle By Name(w653) -> ("跨度核查数据时间"=w652:timestamp, "跨度核查实测值"=w651:sgl, "跨度核查数据标识"=w650:string)
                n177 = Unbundle By Name(w648) -> ("硫化物跨度标准液浓度"=w647:dbl)
              }
              frame "零点核查" {
                n178 = Unbundle By Name(w660) -> ("零点核查数据时间"=w659:timestamp, "零点核查实测值"=w658:sgl, "零点核查数据标识"=w657:string)
                n179 = Unbundle By Name(w655) -> ("硫化物零点标准液浓度"=w654:dbl)
              }
              frame "加标回收" {
                n180 = Unbundle By Name(w665) -> ("加标回收数据时间"=w664:timestamp, "加标回收实测值"=w663:sgl, "加标回收数据标识"=w662:string)
              }
              frame "空白测试" {
                n181 = Unbundle By Name(w670) -> ("空白数据时间"=w669:timestamp, "空白实测值"=w668:sgl, "空白数据标识"=w667:string)
              }
              frame "平行样" {
                n182 = Unbundle By Name(w675) -> ("平行样数据时间"=w674:timestamp, "平行样实测值"=w673:sgl, "平行样数据标识"=w672:string)
              }
            }
            n183 = Unbundle By Name(w606) -> ("硫化物跨度值"=w605:dbl)
            n184 = And(x=w612, y=u16 255) -> (x .and. y?=w613:u16)
            n185 = case shown="0, 默认" w613 {
              tunnel: ["低量程" ("格式字符串") "高量程" ("格式字符串")] -> w611
              frame 0, Default {
              }
              frame 1 {
              }
            }
            n186 = global read "VAR总磷总氮全局变量.vi" "序列号"() -> (w610:string)
            n187 = Bundle By Name(cluster=w607, "时间标识"=w618, "监测值"=w617, "数据标识"=w616, "测量模式"=w608, "单位"=w632, "因子编码"=w631, "标样参考值"=w615, "F0"=w630, "F1"=w629, "F2"=w628, "F3"=w627, "F4"=w626, "F5"=w625, "F6"=w624, "F7"=w623, "X"=w622, "温度"=w621, "湿度"=w620, "量程标识"=w611, "SN"=w610, "数据标记表"=w609, "跨度值"=w605, "X1"=w598) -> (w603:T2)
            n188 = global read "VAR总磷总氮全局变量.vi" "硫化物关键参数"() -> (w599:T10)
            n189 = call "总磷氨氮插入数据.vi"("table"=w602, "关键参数"=w599, "data"=w603) -> ()  [unwired: 12 in, 1 out]
          }
          frame 22 {
            n190 = Unbundle By Name(w681) -> ("单位"=w710:u16, "因子编码"=w709:u32, "F0"=w708:sgl, "F1"=w707:sgl, "F2"=w706:sgl, "F3"=w705:sgl, "F4"=w704:sgl, "F5"=w703:sgl, "F6"=w702:sgl, "F7"=w701:sgl, "X值"=w700:sgl, "温度"=w699:sgl, "湿度"=w698:sgl, "fidrange"=w690:u16, "X1值"=w676:sgl)  [unwired: 1 out]
            n191 = global read "总磷总氮断电保存全局变量.vi" "质控参数设置"() -> (w683:T9)
            n192 = case shown="\"标样核查\"" w697 {
              tunnel: w681 -> [w717 w724 w731 w738 w743 w748 w753]
              tunnel: [w716 w723 w730 w737 w742 w747 w752] -> w696
              tunnel: [w715 w722 w729 w736 w741 w746 w751] -> w695
              tunnel: [w714 w721 w728 w735 w740 w745 w750] -> w694
              tunnel: [T4."水样测试" ("测量模式") w718 T4."跨度核查" ("测量模式") T4."零点核查" ("测量模式") T4."加标回收" ("测量模式") w744 T4."平行样测试" ("测量模式")] -> w686
              tunnel: w683 -> [_ w720 w726 w733 _ _ _]
              tunnel: [_ w719 w725 w732 _ _ _] -> w693
              tunnel: w679 -> [_ _ _ _ _ w744 _]
              tunnel: w678 -> [_ w718 _ _ _ _ _]
              frame "水样测试", Default {
                n193 = Unbundle By Name(w717) -> ("水样数据时间"=w716:timestamp, "水样实测值"=w715:sgl, "水样数据标识"=w714:string)
              }
              frame "标样核查" {
                n194 = Unbundle By Name(w724) -> ("标样数据时间"=w723:timestamp, "标样实测值"=w722:sgl, "标样数据标识"=w721:string)
                n195 = Unbundle By Name(w720) -> ("COD标准液标准浓度"=w719:dbl)
              }
              frame "跨度核查" {
                n196 = Unbundle By Name(w731) -> ("跨度核查数据时间"=w730:timestamp, "跨度核查实测值"=w729:sgl, "跨度核查数据标识"=w728:string)
                n197 = Unbundle By Name(w726) -> ("COD跨度标准液浓度"=w725:dbl)
              }
              frame "零点核查" {
                n198 = Unbundle By Name(w738) -> ("零点核查数据时间"=w737:timestamp, "零点核查实测值"=w736:sgl, "零点核查数据标识"=w735:string)
                n199 = Unbundle By Name(w733) -> ("COD零点标准液浓度"=w732:dbl)
              }
              frame "加标回收" {
                n200 = Unbundle By Name(w743) -> ("加标回收数据时间"=w742:timestamp, "加标回收实测值"=w741:sgl, "加标回收数据标识"=w740:string)
              }
              frame "空白测试" {
                n201 = Unbundle By Name(w748) -> ("空白数据时间"=w747:timestamp, "空白实测值"=w746:sgl, "空白数据标识"=w745:string)
              }
              frame "平行样" {
                n202 = Unbundle By Name(w753) -> ("平行样数据时间"=w752:timestamp, "平行样实测值"=w751:sgl, "平行样数据标识"=w750:string)
              }
            }
            n203 = Unbundle By Name(w683) -> ("COD跨度值"=w682:dbl)
            n204 = And(x=w690, y=u16 255) -> (x .and. y?=w691:u16)
            n205 = case shown="0, 默认" w691 {
              tunnel: ["低量程" ("格式字符串") "高量程" ("格式字符串")] -> w689
              frame 0, Default {
              }
              frame 1 {
              }
            }
            n206 = global read "VAR总磷总氮全局变量.vi" "序列号"() -> (w688:string)
            n207 = Bundle By Name(cluster=w685, "时间标识"=w696, "监测值"=w695, "数据标识"=w694, "测量模式"=w686, "单位"=w710, "因子编码"=w709, "标样参考值"=w693, "F0"=w708, "F1"=w707, "F2"=w706, "F3"=w705, "F4"=w704, "F5"=w703, "F6"=w702, "F7"=w701, "X"=w700, "温度"=w699, "湿度"=w698, "量程标识"=w689, "SN"=w688, "数据标记表"=w687, "跨度值"=w682, "X1"=w676) -> (w684:T2)
            n208 = global read "VAR总磷总氮全局变量.vi" "CODcr关键参数"() -> (w677:T10)
            n209 = call "总磷氨氮插入数据.vi"("table"=w680, "关键参数"=w677, "data"=w684) -> ()  [unwired: 12 in, 1 out]
          }
        }
      }
    }
  }
